vi "Initialise.vi"() -> (3 "EEPROM out":refnum<class "EEPROM.lvclass">)   [LabVIEW 2021, in "EEPROM.lvclass"]
uses:
  EEPROM.lvclass
  EEPROM.lvclass/EEPROM.ctl
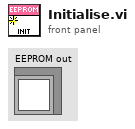
[diagram p1: front panel]
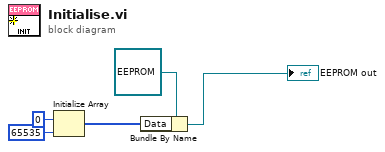
[diagram p0: block diagram]
diagram:
  n1 = Initialize Array(u8 0 ("element"), 65535 ("dimension size")) -> (w2:u8[])
  n2 = Bundle By Name(cluster=refnum<class "EEPROM.lvclass"> refnum ("EEPROM in"), "Data"=w2) -> (→"EEPROM out":refnum<class "EEPROM.lvclass">)
